vi "Reset CAN Device.vi"(8 "error in (no error)":errorcluster, 11 "Cluster in":refnum<vi>) -> (0 "error out":errorcluster)   [LabVIEW 2017]
uses:
  PCAN_Driver/ControlCAN.lvlib
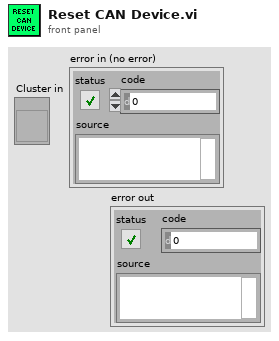
[diagram p1: front panel]
types:
  T1 = typedef "ControlCAN.lvlib/DevType.ctl" = u32
  T2 = typedef "ControlCAN.lvlib/CAN Channel.ctl" = u32
  T3 = typedef "ControlCAN.lvlib/VCI_INIT_CONFIG.ctl" = cluster{"AccCode":u32, "AccMask":u32, "InitFlag":T4, "Fliter":T5, "Timing0":u8, "Timing1":u8, "Mode":T6}
  T4 = typedef "ControlCAN.lvlib/InitFlag.ctl" = u32
  T5 = typedef "ControlCAN.lvlib/Fliter.ctl" = u8
  T6 = typedef "ControlCAN.lvlib/Mode.ctl" = u8
  T7 = cluster{"DevType":T1, "DevIndex":u32, "CanIndex":T2, "VCI_INIT_CONFIG":T3}
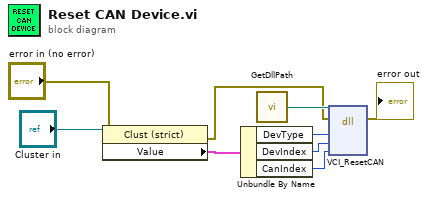
[diagram p0: block diagram]
diagram:
  n1 = property class="Clust (strict)"(reference="Cluster in", error in="error in (no error)") -> (error out=w2:errorcluster, "Value"=w6:T7)  [unwired: 1 out]
  n2 = Unbundle By Name(w6) -> ("DevType"=w7:T1, "DevIndex"=w8:u32, "CanIndex"=w4:T2)
  n3 = call "GetDllPath.vi"() -> ("DllPath"=w5:path)  [unwired: 1 in]
  n4 = dll-call lib="C:/Projects/Marvin CAN UTD/MarvinATP/data/ControlCAN.dll" fn="VCI_ResetCAN"(path in=w5, error in=w2, "DevType"=w7, "DevIndex"=w8, "CANIndex"=w4) -> (error out=→"error out":errorcluster)  [unwired: 5 in, 1 out]
